vi "Holding Register Set Starting Address.vi"(8 "error in (no error)":errorcluster, 10 "Value":u16, 11 "Item Ref in":T1 format="%.0x") -> (0 "error out":errorcluster, 3 "Item Ref out":T1 format="%.0x")   [LabVIEW 2015, in "Modbus Master System Explorer.lvlib"]
uses:
  Modbus Master System Explorer.lvlib
  <vilib>/NI Veristand/Custom Device API/Custom Device Item Ref.ctl
  Shared/Constants.vi
  <vilib>/NI Veristand/Custom Device API/Set Item Property (U16).vi
  <vilib>/NI VeriStand/Custom Device API/Custom Device API.lvlib
  Shared/Modbus Master Shared.lvlib
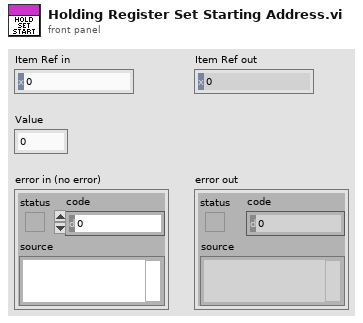
[diagram p1: front panel]
types:
  T1 = typedef "Custom Device API.lvlib/Custom Device Item Ref.ctl" = u64
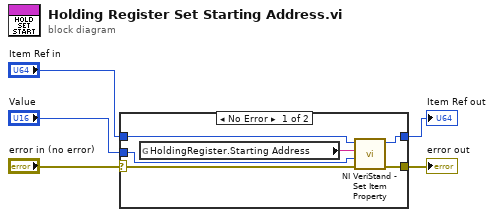
[diagram p0: block diagram]
diagram:
  n1 = case shown="No Error" "error in (no error)" {
    selector: "error in (no error)" -> [w10 w12]
    tunnel: "Item Ref in" -> [w9 w13]
    tunnel: [w8 w12] -> w3
    tunnel: [w7 w13] -> w2
    tunnel: "Value" -> [w6 _]
    frame No Error {
      n2 = global read "Constants.vi" "HoldingRegister.Starting Address"() -> (w11:string)
      n3 = call-poly <vilib>:"NI VeriStand - Set Item Property.vi"("error in (no error)"=w10, "Value"=w6, "Property Name"=w11, "Item Ref in"=w9) -> ("error out"=w8:errorcluster, "Item Ref out"=w7:T1)  [unwired: 5 in, 1 out]
    }
    frame Error {
    }
  }
  "error out" <- w3
  "Item Ref out" <- w2
